vi "Default CDO Channels.vi"(1 "Channels":T3={"# Input Channels"=0, "# Output Channels"=0, "Channel Type"=enum."Digital", "Units"=""}) -> (0 "CDO":T1)   [LabVIEW 2020, in "Modules.lvlib" / "SD Module.lvclass"]
uses:
  SD Module.lvclass
  RSI Module/Channels.ctl
  RSI Module/Channel Type.ctl
  Type Defs/CDO.ctl
  Type Defs/CDO Channel.ctl
  RSI Module/RSI Module.lvclass
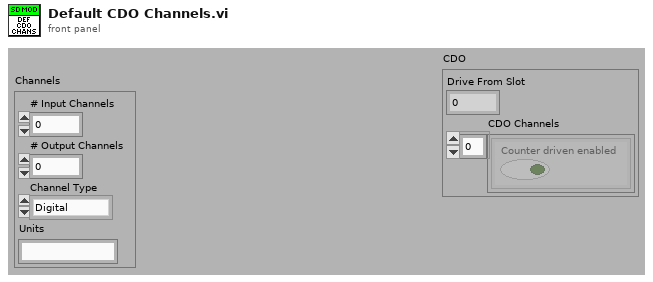
[diagram p1: front panel]
types:
  T1 = typedef "Modules.lvlib/SD Module.lvclass/CDO.ctl" = cluster{"Drive From Slot":u32, "CDO Channels":T2[]}
  T2 = typedef "Modules.lvlib/SD Module.lvclass/CDO Channel.ctl" = cluster{"Counter driven enabled":bool}
  T3 = typedef "Modules.lvlib/RSI Module.lvclass/Channels.ctl" = cluster{"# Input Channels":i32, "# Output Channels":i32, "Channel Type":T4, "Units":string}
  T4 = typedef "Modules.lvlib/RSI Module.lvclass/Channel Type.ctl" = enum16{"Analog", "Digital"}
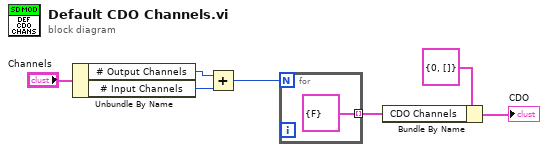
[diagram p0: block diagram]
diagram:
  n1 = Unbundle By Name("Channels") -> ("# Output Channels"=w3:i32, "# Input Channels"=w2:i32)
  n2 = Add(x=w3, y=w2) -> (x+y=w1:i32)
  n3 = for {
    N: w1 -> [_]
    tunnel: [T2 {"Counter driven enabled"=FALSE} ("CDO Channel")] -> w4 mode=indexing
  }
  n4 = Bundle By Name(cluster=T1 {"Drive From Slot"=0, "CDO Channels"=[]} ("CDO"), "CDO Channels"=w4) -> (→"CDO":T1)
